vi "write driver inputs.vi"(0 "Jx":dbl, 1 "Jy":dbl, 2 "Jr":dbl, 8 "stack prefix":string) -> ()   [LabVIEW 2023]
uses:
  <vilib>/Rock Robotics/Network Tables/NT Write Number.vi
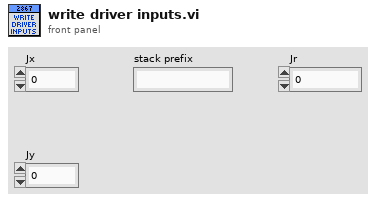
[diagram p1: front panel]
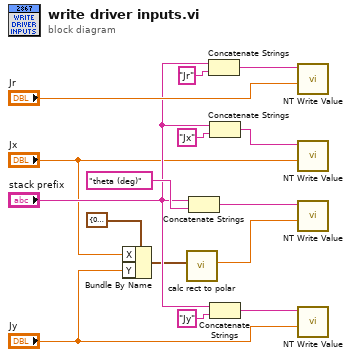
[diagram p0: block diagram]
diagram:
  n1 = Bundle By Name(cluster=cluster{"X":dbl, "Y":dbl} {"X"=0.0, "Y"=0.0} ("XY"), "X"="Jx", "Y"="Jy") -> (w4:cluster{"X":dbl, "Y":dbl})
  n2 = call "calc rect to polar.vi"("XY"=w4) -> ("angle (deg)"=w1:dbl)  [unwired: 8 in, 2 out]
  n3 = Concatenate Strings("stack prefix", "theta (deg)" ("string")) -> (w14:string)
  n4 = Concatenate Strings("stack prefix", "Jr" ("string")) -> (w13:string)
  n5 = Concatenate Strings("stack prefix", "Jx" ("string")) -> (w11:string)
  n6 = Concatenate Strings("stack prefix", "Jy" ("string")) -> (w12:string)
  n7 = call-poly <vilib>:"NT Write Value.vi"("value"="Jr", "name"=w13) -> ()  [unwired: 9 in, 1 out]
  n8 = call-poly <vilib>:"NT Write Value.vi"("value"="Jx", "name"=w11) -> ()  [unwired: 9 in, 1 out]
  n9 = call-poly <vilib>:"NT Write Value.vi"("value"=w1, "name"=w14) -> ()  [unwired: 9 in, 1 out]
  n10 = call-poly <vilib>:"NT Write Value.vi"("value"="Jy", "name"=w12) -> ()  [unwired: 9 in, 1 out]
